vi "main_GBATP_Sample.vi"() -> ()   [LabVIEW 2020]
panel:
  in  "Stop Button":bool
  in  "Setting Tab":T1(tab)
  in  "file path (dialog if empty)":path=path "C:/Users/user/Desktop/AutoSampler/AutoSampler _GB/ATP.txt"
  in  "start of read offset (chars.:0)":i32
  in  "max characters/row  (no limit:0)":i32
  out "mark after read (chars.)":i32=406
  in  "number of rows (all:-1)":i32=-1
  out "all rows":string[][](array[string])=[["58"], ["257"], ["0"], ["0"], ["58"], ["257"], ["100"], ["50"], ["58"], ["257"], ["0"], ["50"], ["58"], ["470"], ["0"], ["50"], ["58"], ["470"], ["100"], ["0"], ["58"], ["470"], ["0"], ["0"], ["120"], ["470"], ["0"], ["0"], ["120"], ["470"], ["100"], ["50"], ["120"], ["470"], ["0"], ["50"], ["120"], ["550"], ["0"], ["50"], ["120"], ["550"], ["100"], ["0"], ["120"], ["550"], ["0"], ["0"], ["120"], ["470"], ["0"], ["0"], ["120"], ["470"], ["100"], ["50"], ["120"], ["470"], ["0"], ["50"], ["120"], ["550"], ["0"], ["50"], ["120"], ["550"], ["100"], ["0"], ["120"], ["550"], ["0"], ["0"], ["120"], ["470"], ["0"], ["0"], ["120"], ["470"], ["100"], ["50"], ["120"], ["470"], ["0"], ["50"], ["120"], ["550"], ["0"], ["50"], ["120"], ["550"], ["100"], ["0"], ["120"], ["550"], ["0"], ["0"]]
  in  "format (%.3f)":string="%.3f"
  in  "transpose (no:F)":bool
  in  "type (empty)":string[][](array[string])
  in  "delimiter (Tab)":string="\t"
  out "EOF?":bool
  out "Size(s)":i32=96
  in  "Sampling Measurement Time(S)":dbl=10.0
  out "X, Y, Z, S":i32
  out "Index":i32=180
  out "Value":string="58"
  out "Current Position(mm)":dbl
  out "Arrived":bool=TRUE
  in  "Occupied Length by Air(mm)":dbl format="%#_13g"
  out "Even Number":dbl=1.0
  out "Action":bool=TRUE
  out "Current Time Index":i32=20
  out "Index 2":i32=180
  in  "file path (dialog if empty) 2":path=path "C:/Users/user/Desktop/AutoSampler/AutoSampler _GB/SamplePosition.txt"
  in  "start of read offset (chars.:0) 2":i32
  in  "max characters/row  (no limit:0) 2":i32
  out "mark after read (chars.) 2":i32=1632
  in  "number of rows (all:-1) 2":i32=-1
  out "all rows 2":string[][](array[string])=[["58"], ["257"], ["0"], ["0"], ["58"], ["257"], ["100"], ["0"], ["58"], ["257"], ["0"], ["0"], ["58"], ["0"], ["0"], ["0"], ["58"], ["0"], ["100"], ["0"], ["58"], ["0"], ["0"], ["0"], ["120"], ["470"], ["0"], ["0"], ["120"], ["470"], ["100"], ["0"], ["120"], ["470"], ["0"], ["0"], ["120"], ["550"], ["0"], ["0"], ["120"], ["550"], ["100"], ["0"], ["120"], ["550"], ["0"], ["0"], ["120"], ["470"], ["0"], ["0"], ["120"], ["470"], ["100"], ["0"], ["120"], ["470"], ["0"], ["0"], ["120"], ["550"], ["0"], ["0"], ["120"], ["550"], ["100"], ["0"], ["120"], ["550"], ["0"], ["0"], ["120"], ["470"], ["0"], ["0"], ["120"], ["470"], ["100"], ["0"], ["120"], ["470"], ["0"], ["0"], ["120"], ["550"], ["0"], ["0"], ["120"], ["550"], ["100"], ["0"], ["120"], ["550"], ["0"], ["0"], ["58"], ["257"], ["0"], ["0"], ["58"], ["257"], ["100"], ["0"], ["58"], ["257"], ["0"], ["0"], ["58"], ["9"], ["0"], ["0"], ["58"], ["9"], ["100"], ["0"], ["58"], ["9"], ["0"], ["0"], ["120"], ["470"], ["0"], ["0"], ["120"], ["470"], ["100"], ["0"], ["120"], ["470"], ["0"], ["0"], ["120"], ["550"], ["0"], ["0"], ["120"], ["550"], ["100"], ["0"], ["120"], ["550"], ["0"], ["0"], ["120"], ["470"], ["0"], ["0"], ["120"], ["470"], ["100"], ["0"], ["120"], ["470"], ["0"], ["0"], ["120"], ["550"], ["0"], ["0"], ["120"], ["550"], ["100"], ["0"], ["120"], ["550"], ["0"], ["0"], ["58"], ["18"], ["0"], ["0"], ["58"], ["18"], ["100"], ["0"], ["58"], ["18"], ["0"], ["0"], ["58"], ["27"], ["0"], ["0"], ["58"], ["27"], ["100"], ["0"], ["58"], ["27"], ["0"], ["0"], ["58"], ["36"], ["0"], ["0"], ["58"], ["36"], ["100"], ["0"], ["58"], ["36"], ["0"], ["0"], ["58"], ["45"], ["0"], ["0"], ["58"], ["45"], ["100"], ["0"], ["58"], ["45"], ["0"], ["0"], ["58"], ["54"], ["0"], ["0"], ["58"], ["54"], ["100"], ["0"], ["58"], ["54"], ["0"], ["0"], ["58"], ["63"], ["0"], ["0"], ["58"], ["63"], ["100"], ["0"], ["58"], ["63"], ["0"], ["0"], ["49"], ["63"], ["0"], ["0"], ["49"], ["63"], ["100"], ["0"], ["49"], ["63"], ["0"], ["0"], ["49"], ["54"], ["0"], ["0"], ["49"], ["54"], ["100"], ["0"], ["49"], ["54"], ["0"], ["0"], ["49"], ["45"], ["0"], ["0"], ["49"], ["45"], ["100"], ["0"], ["49"], ["45"], ["0"], ["0"], ["49"], ["36"], ["0"], ["0"], ["49"], ["36"], ["100"], ["0"], ["49"], ["36"], ["0"], ["0"], ["49"], ["27"], ["0"], ["0"], ["49"], ["27"], ["100"], ["0"], ["49"], ["27"], ["0"], ["0"], ["49"], ["18"], ["0"], ["0"], ["49"], ["18"], ["100"], ["0"], ["49"], ["18"], ["0"], ["0"], ["49"], ["9"], ["0"], ["0"], ["49"], ["9"], ["100"], ["0"], ["49"], ["9"], ["0"], ["0"], ["49"], ["0"], ["0"], ["0"], ["49"], ["0"], ["100"], ["0"], ["49"], ["0"], ["0"], ["0"], ["40"], ["0"], ["0"], ["0"], ["40"], ["0"], ["100"], ["0"], ["40"], ["0"], ["0"], ["0"], ["40"], ["9"], ["0"], ["0"], ["40"], ["9"], ["100"], ["0"], ["40"], ["9"], ["0"], ["0"], ["40"], ["18"], ["0"], ["0"], ["40"], ["18"], ["100"], ["0"], ["40"], ["18"], ["0"], ["0"], ["40"], ["27"], ["0"], ["0"], ["40"], ["27"], ["100"], ["0"], ["40"], ["27"], ["0"], ["0"], ["40"], ["36"], ["0"], ["0"], ["40"], ["36"], ["100"], ["0"], ["40"], ["36"], ["0"], ["0"], ["40"], ["45"], ["0"], ["0"], ["40"], ["45"], ["100"], ["0"], ["40"], ["45"], ["0"], ["0"], ["40"], ["54"], ["0"], ["0"], ["40"], ["54"], ["100"], ["0"], ["40"], ["54"], ["0"], ["0"], ["40"], ["63"], ["0"], ["0"], ["40"], ["63"], ["100"], ["0"], ["40"], ["63"], ["0"], ["0"]]
  in  "format (%.3f) 2":string="%.3f"
  in  "transpose (no:F) 2":bool
  in  "type (empty) 2":string[][](array[string])
  in  "delimiter (Tab) 2":string="\t"
  out "EOF? 2":bool
  out "Size(s) 2":i32=432
  out "error out":errorcluster={"status"=FALSE, "code"=1073676294, "source"="VISA Read in position_read.vi->main_GB01.vi"}
  out "S Connecting":bool
  out "Z Connecting":bool
  out "Y Connecting":bool
  out "X  Connecting":bool
  in  "COM Port":refnum<visa-resource-name>="COM3"
  # "Position :"
  # "(set the Occupied length by Air if the target axis is syringe axis)"
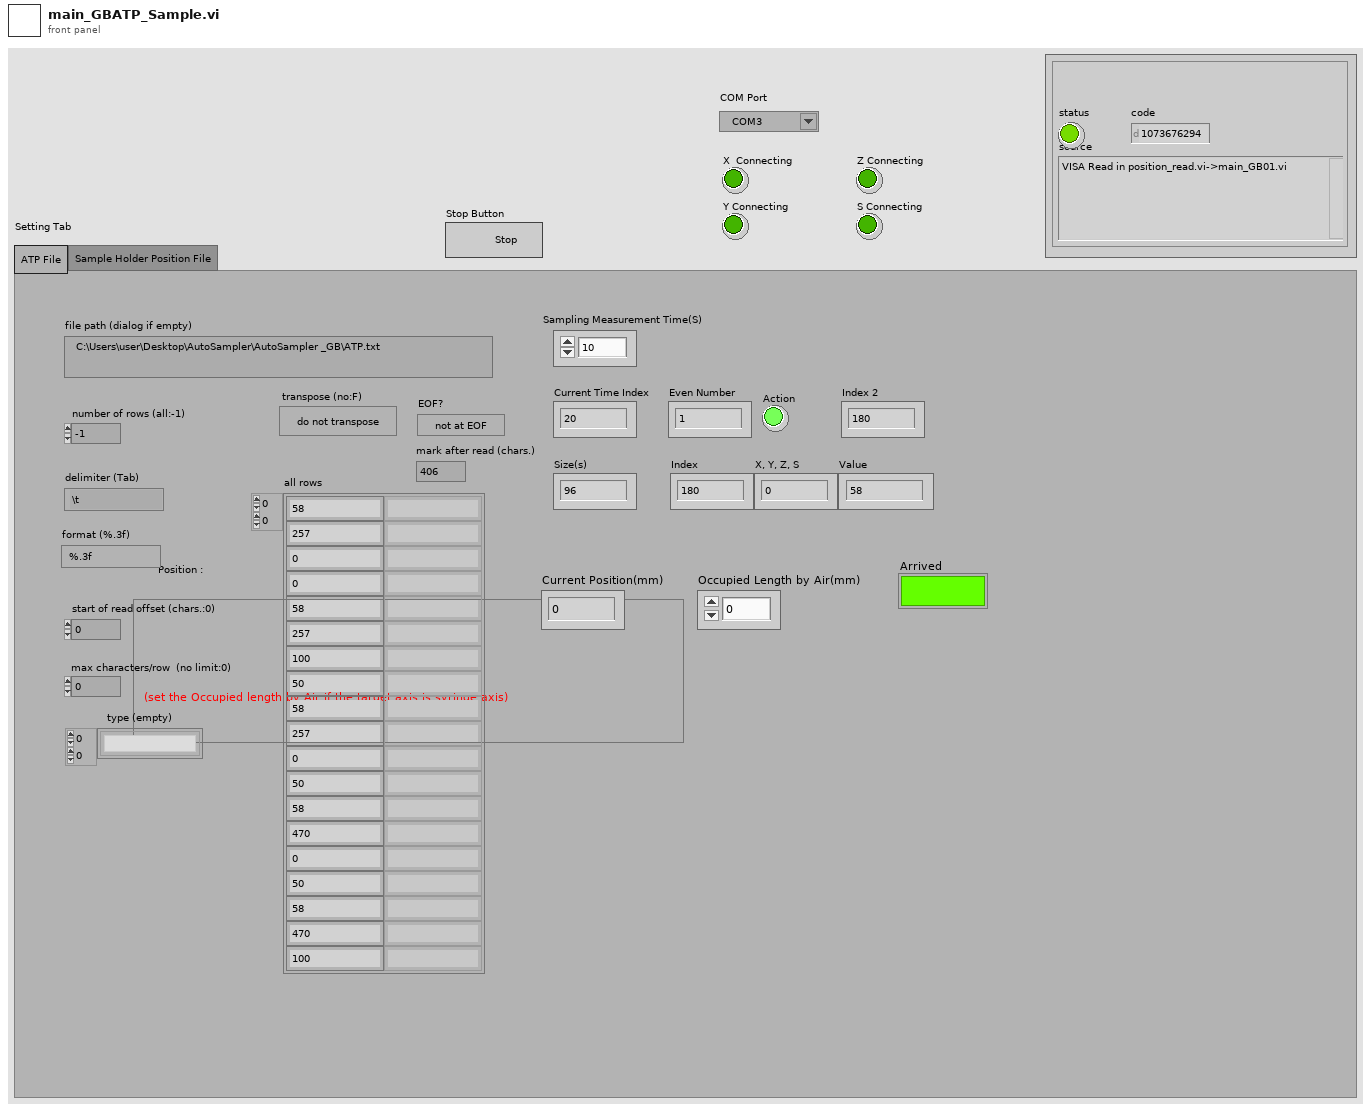
[diagram p1: front panel]
types:
  T1 = enum32{"ATP File", "Sample Holder Position File"}
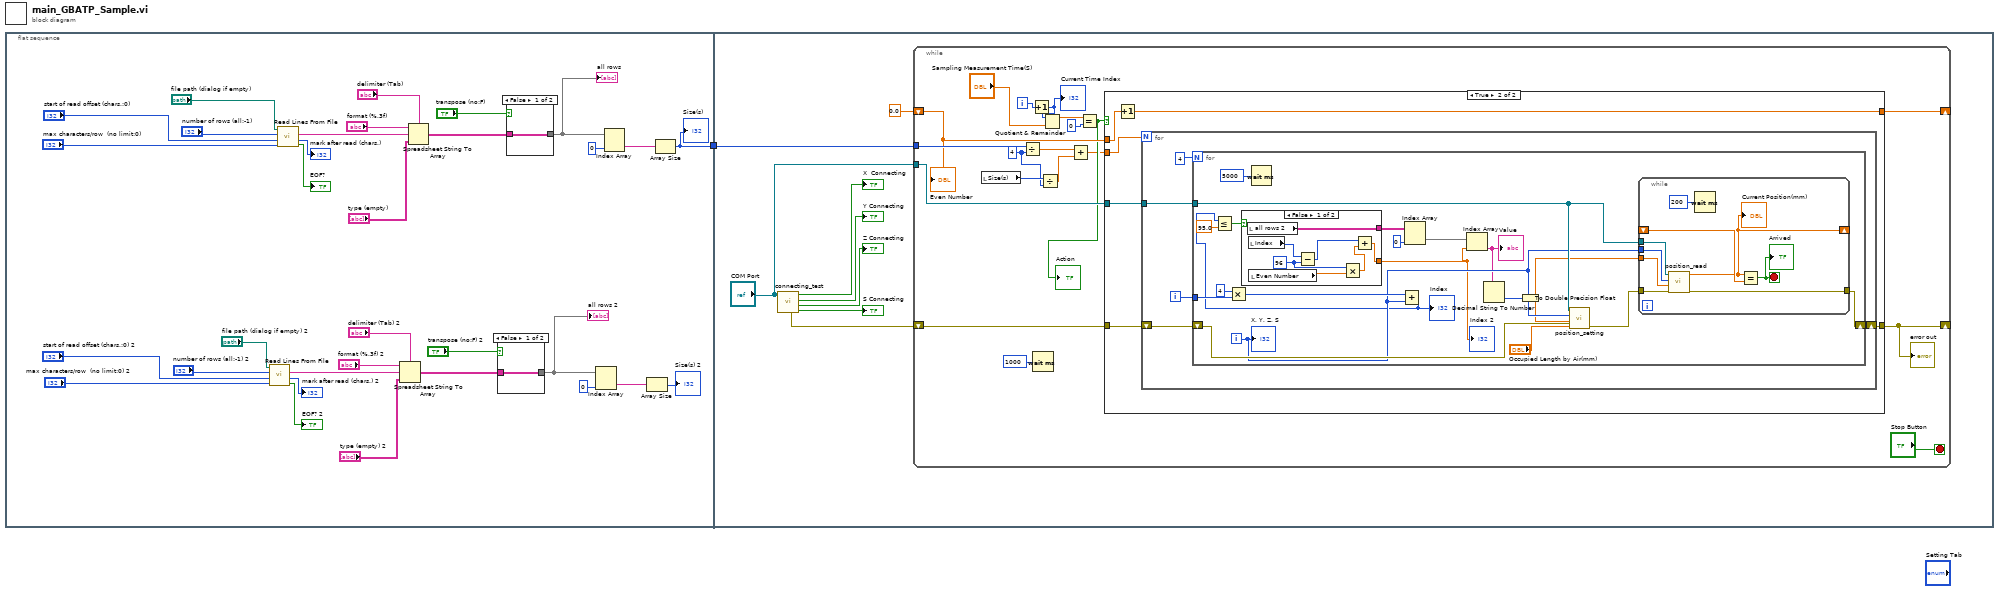
[diagram p0: block diagram]
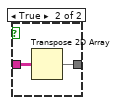
[diagram p2: hidden frame]
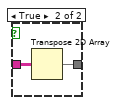
[diagram p3: hidden frame]
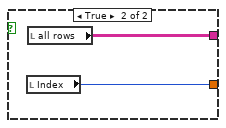
[diagram p5: hidden frame]
diagram:
  n1 = flat-sequence {
    tunnel: [w19] -> w1
    tunnel: w1 -> [w41]
    frame #0 {
      n2 = call <vilib>:"Read Lines From File.vi"("file path (dialog if empty)"="file path (dialog if empty) 2", "number of lines (all:-1)"="number of rows (all:-1) 2", "start of read offset (chars.:0)"="start of read offset (chars.:0) 2", "[max characters per line]  (no limit:0)"="max characters/row  (no limit:0) 2") -> ("line string"=w14:string, "mark after read (chars.)"=→"mark after read (chars.) 2":i32, "EOF?"=→"EOF? 2":bool)  [unwired: 2 in, 1 out]
      n3 = call <vilib>:"Read Lines From File.vi"("file path (dialog if empty)"="file path (dialog if empty)", "number of lines (all:-1)"="number of rows (all:-1)", "start of read offset (chars.:0)"="start of read offset (chars.:0)", "[max characters per line]  (no limit:0)"="max characters/row  (no limit:0)") -> ("line string"=w29:string, "mark after read (chars.)"=→"mark after read (chars.)":i32, "EOF?"=→"EOF?":bool)  [unwired: 2 in, 1 out]
      n4 = Spreadsheet String To Array(delimiter (Tab)="delimiter (Tab) 2", format string="format (%.3f) 2", spreadsheet string=w14, array type (2D Dbl)="type (empty) 2") -> (array=w12:string[][])
      n5 = Spreadsheet String To Array(delimiter (Tab)="delimiter (Tab)", format string="format (%.3f)", spreadsheet string=w29, array type (2D Dbl)="type (empty)") -> (array=w27:string[][])
      n6 = case shown="False" "transpose (no:F) 2" {
        tunnel: [w34 w36] -> w2
        tunnel: w12 -> [w34 w35]
        frame False {
        }
        frame True {
          n7 = Transpose 2D Array(2D array=w35) -> (transposed array=w36:string[][])
        }
      }
      "all rows 2" <- w2
      n8 = case shown="False" "transpose (no:F)" {
        tunnel: [w37 w39] -> w3
        tunnel: w27 -> [w37 w38]
        frame False {
        }
        frame True {
          n9 = Transpose 2D Array(2D array=w38) -> (transposed array=w39:string[][])
        }
      }
      "all rows" <- w3
      n10 = Index Array "Index Array"(array=w2, index (col)=0) -> (element=w5:string[])  [unwired: 1 in]
      n11 = Index Array "Index Array"(array=w3, index (col)=0) -> (element=w20:string[])  [unwired: 1 in]
      n12 = Array Size(array=w5) -> (size(s)=→"Size(s) 2":i32)
      n13 = Array Size(array=w20) -> (size(s)=w19:i32)
      "Size(s)" <- w19
    }
    frame #1 {
      n14 = call "connecting_test.vi"("VISA resource name"="COM Port") -> ("syringe axis connecting"=→"S Connecting":bool, "Z axis connecting"=→"Z Connecting":bool, "Y axis connecting"=→"Y Connecting":bool, "X axis connecting"=→"X  Connecting":bool, "error out"=w44:errorcluster)  [unwired: 6 in]
      n15 = while {
        shift-right: [w65] -> _
        shift-left: w44 -> [w66]
        tunnel: "COM Port" -> [w63]
        tunnel: w41 -> [w59]
        shift-right: [w58] -> _
        shift-left: 0.0 -> [w57]
        i -> [w55]
        stop <- "Stop Button" stop-if-true
        w49 = 4 ("y")
        n16 = local read "Size(s)"() -> (w50:i32)
        n17 = Divide(x=w59, y=w49) -> (x/y=w52:dbl)
        n18 = Increment(x=w55) -> (x+1=w54:i32)
        "Current Time Index" <- w54
        n19 = Wait (ms)(milliseconds to wait=u32 1000) -> ()  [unwired: 1 out]
        n20 = Divide(x=w50, y=w49) -> (x/y=w48:dbl)
        n21 = Quotient & Remainder(x=w54, y="Sampling Measurement Time(S)") -> (x-y*floor(x/y)=w60:dbl)  [unwired: 1 out]
        n22 = Add(x=w52, y=w48) -> (x+y=w51:dbl)
        n23 = Equal?(x=w60, y=0) -> (x = y?=w56:bool)
        "Action" <- w56
        n24 = case shown="True" w56 {
          tunnel: w66 -> [w67 w74]
          tunnel: [w67 w73] -> w65
          tunnel: w63 -> [_ w72]
          tunnel: w57 -> [w68 w70]
          tunnel: [w68 w71] -> w58
          tunnel: w51 -> [_ w69]
          frame False {
          }
          frame True {
            n25 = Increment(x=w70) -> (x+1=w71:dbl)
            n26 = for {
              N: w69 -> [_]
              tunnel: w72 -> [w77]
              shift-right: [w78] -> w73
              shift-left: w74 -> [w79]
              i -> [w75]
              n27 = for {
                N: 4 -> [_]
                tunnel: w77 -> [w95]
                shift-right: [w98] -> w78
                shift-left: w79 -> [w99]
                tunnel: w75 -> [w84]
                i -> [w92]
                n28 = Multiply(x=4, y=w84) -> (x*y=w94:i32)
                n29 = Wait (ms)(milliseconds to wait=u32 5000) -> ()  [unwired: 1 out]
                n30 = Add(x=w94, y=w92) -> (x+y=w81:i32)
                "Index" <- w81
                n31 = Less Or Equal?(x=w81, y=95.0) -> (x <= y?=w83:bool)
                n32 = case shown="False" w83 {
                  tunnel: [w106 w108] -> w90
                  tunnel: [w101 w107] -> w80
                  frame False {
                    w104 = 96 ("y")
                    n33 = local read "all rows 2"() -> (w106:string[][])
                    n34 = local read "Index"() -> (w105:i32)
                    n35 = local read "Even Number"() -> (w100:dbl)
                    n36 = Subtract(x=w105, y=w104) -> (x-y=w103:i32)
                    n37 = Multiply(x=w104, y=w100) -> (x*y=w102:dbl)
                    n38 = Add(x=w103, y=w102) -> (x+y=w101:dbl)
                  }
                  frame True {
                    n39 = local read "Index"() -> (w107:i32)
                    n40 = local read "all rows"() -> (w108:string[][])
                  }
                }
                "Index 2" <- w80
                n41 = Index Array "Index Array"(array=w90, index (col)=0) -> (element=w91:string[])  [unwired: 1 in]
                n42 = Index Array(array=w91, index=w80) -> (element=w88:string)
                "Value" <- w88
                n43 = Decimal String To Number(string=w88) -> (number=w86:i32)  [unwired: 2 in, 1 out]
                n44 = To Double Precision Float(number=w86) -> (double precision float=w85:dbl)
                n45 = call "position_setting.vi"("error in (no error)"=w99, "Occupied length by Air(mm)"="Occupied Length by Air(mm)", "Distance(mm)"=w85, "Axis"=w92, "Com Port"=w95) -> ("error out"=w97:errorcluster)  [unwired: 6 in]
                n46 = while {
                  tunnel: w92 -> [w117]
                  tunnel: w85 -> [w116]
                  tunnel: [w115] -> w98
                  tunnel: w97 -> [w114]
                  shift-right: [w112] -> _
                  shift-left: _ -> [w113]
                  tunnel: w95 -> [w109]
                  stop <- w110 stop-if-true
                  n47 = call "position_read.vi"("error in (no error)"=w114, "Occupied Length by Air(mm)"=w116, "Axis"=w117, "COM Port"=w109) -> ("error out"=w115:errorcluster, "current position(mm)"=w112:dbl)  [unwired: 6 in]
                  "Current Position(mm)" <- w112
                  n48 = Wait (ms)(milliseconds to wait=u32 200) -> ()  [unwired: 1 out]
                  n49 = Equal?(x=w112, y=w113) -> (x = y?=w110:bool)
                  "Arrived" <- w110
                }
                "X, Y, Z, S" <- w92
              }
            }
          }
        }
        "error out" <- w65
        "Even Number" <- w57
      }
    }
  }
